vi "Stop FP Server.vi"(8 "error in (no error)":errorcluster, 10 "Timeout (-1)":i32=-1, 11 "FP Management In":refnum<class "Front Panel Manager.lvclass">) -> (0 "error out":errorcluster, 3 "FP Management Out":refnum<class "Front Panel Manager.lvclass">)   [LabVIEW 2015, in "Front Panel Publisher.lvlib" / "Front Panel Manager.lvclass"]
uses:
  Front Panel Manager.lvclass
  FP Server Message.ctl
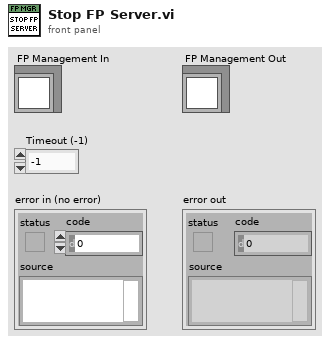
[diagram p1: front panel]
types:
  T1 = enum16{"ReadRepository", "CreateNew", "CreateOrLookUpExisting", "ReadRepositoryAndDestroy"}
  T2 = typedef "Front Panel Publisher.lvlib/Front Panel Manager.lvclass/FP Server Message.ctl" = cluster{"Message":string, "Page":string, "Data":string[][], "Connection ID":u64, "Values and Position":refnum<vi>[]}
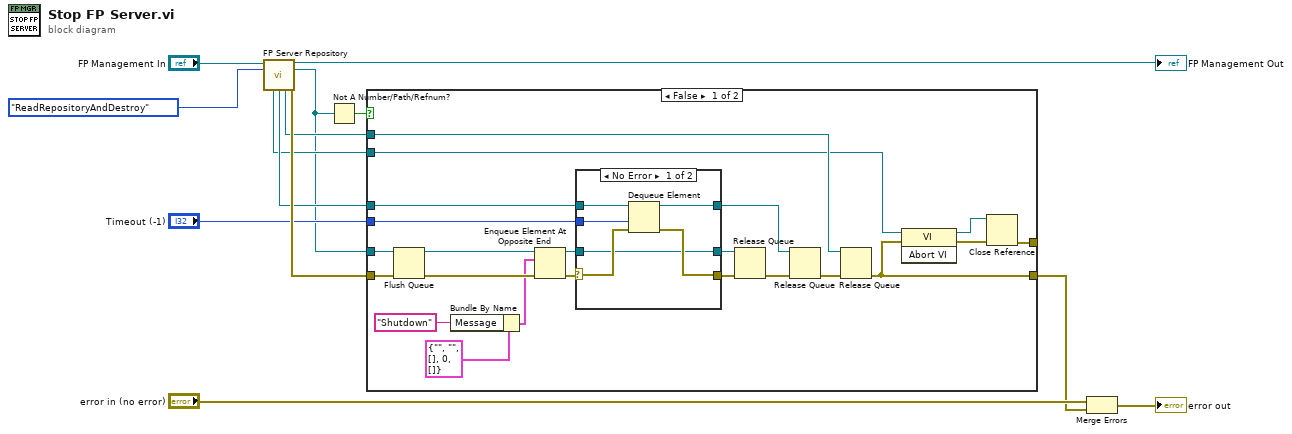
[diagram p0: block diagram]
diagram:
  n1 = call "FP Server Repository.vi"("FP Management In"="FP Management In", "Action(ReadRepository)"=T1."ReadRepositoryAndDestroy") -> ("FP Management Out"=→"FP Management Out":refnum<class "Front Panel Manager.lvclass">, "ToProcessQueue"=w3:refnum<queue>, "ProcessViRef"=w4:refnum<vi>, "ProcessSyncQueue"=w6:refnum<queue>, "FromProcessQueue"=w5:refnum<queue>, "error out"=w10:errorcluster)  [unwired: 7 in, 1 out]
  n2 = Not A Number/Path/Refnum?(number/path/refnum=w3) -> (NaN/Path/Refnum?=w2:bool)
  n3 = case shown="False" w2 {
    tunnel: w6 -> [w24 _]
    tunnel: w10 -> [w34 w45]
    tunnel: [w28 w45] -> w12
    tunnel: w3 -> [w26 _]
    tunnel: "Timeout (-1)" -> [w21 _]
    tunnel: w5 -> [w20 _]
    tunnel: w4 -> [w18 _]
    tunnel: [w27 _] -> _
    frame False {
      n4 = Flush Queue(queue=w26, error in (no error)=w34) -> (queue out=w25:refnum<queue>, error out=w35:errorcluster)  [unwired: 1 out]
      n5 = Bundle By Name(cluster=T2 {"Message"="", "Page"="", "Data"=[], "Connection ID"=0, "Values and Position"=[]} ("Process Message"), "Message"="Shutdown" ("element")) -> (w15:T2)
      n6 = Enqueue Element At Opposite End(queue=w25, element=w15, error in (no error)=w35) -> (queue out=w23:refnum<queue>, error out=w32:errorcluster)  [unwired: 1 in, 1 out]
      n7 = case shown="No Error" w32 {
        tunnel: [w40 w44] -> w33
        tunnel: w24 -> [w38 w42]
        tunnel: [w39 w43] -> w22
        tunnel: w23 -> [w39 w43]
        tunnel: w21 -> [w37 _]
        selector: w32 -> [w41 w44]
        tunnel: [w36 w42] -> w19
        frame No Error {
          n8 = Dequeue Element(queue=w38, timeout in ms (-1)=w37, error in (no error)=w41) -> (queue out=w36:refnum<queue>, error out=w40:errorcluster)  [unwired: 2 out]
        }
        frame Error {
        }
      }
      n9 = Release Queue(queue=w22, error in (no error)=w33) -> (error out=w31:errorcluster)  [unwired: 1 in, 2 out]
      n10 = Release Queue(queue=w19, error in (no error)=w31) -> (error out=w30:errorcluster)  [unwired: 1 in, 2 out]
      n11 = Release Queue(queue=w20, error in (no error)=w30) -> (error out=w28:errorcluster)  [unwired: 1 in, 2 out]
      n12 = invoke class="VI" method="Abort VI"(reference=w18, error in=w28) -> (reference out=w17:refnum<vi>, error out=w29:errorcluster)  [unwired: 1 in, 1 out]
      n13 = Close Reference(reference=w17, error in (no error)=w29) -> (error out=w27:errorcluster)
    }
    frame True {
    }
  }
  n14 = Merge Errors("error in (no error)", w12) -> (→"error out":errorcluster)
